vi "Init.vi"(8 "error in (no error)":errorcluster, 9 "ExecCtrlRefs":T1) -> (0 "error out":errorcluster, 3 "UI ExecutionCtrls out":refnum<class "UI ExecutionCtrls.lvclass">)   [LabVIEW 2019, in "UI ExecutionCtrls.lvclass"]
doc: "store control refs for updating the UI\ninit controls"
uses:
  UI ExecutionCtrls.lvclass
  MotionExecutionCtrlRefs.ctl
  UI ExecutionCtrls.lvclass/UI ExecutionCtrls.ctl
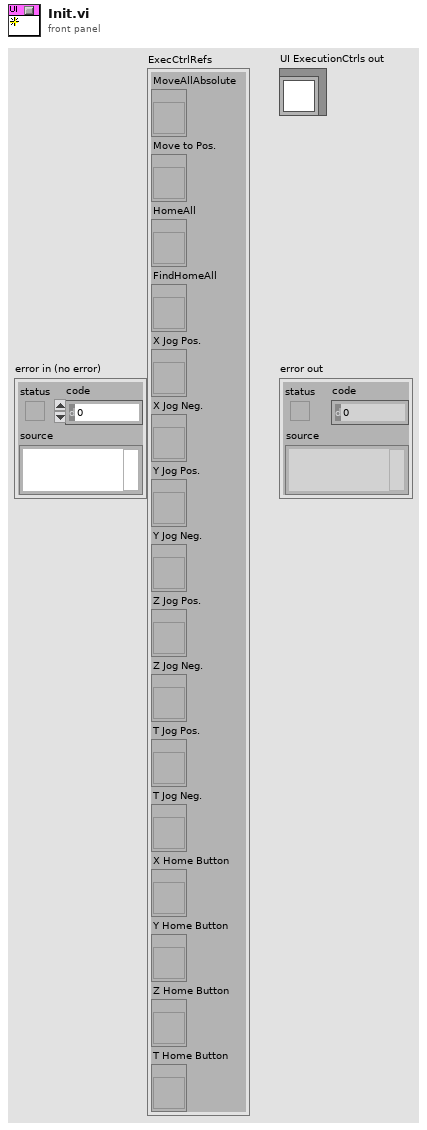
[diagram p1: front panel]
types:
  T1 = typedef "MotionExecutionCtrlRefs.ctl" = cluster{"MoveAllAbsolute":refnum<vi>, "Move to Pos.":refnum<vi>, "HomeAll":refnum<vi>, "FindHomeAll":refnum<vi>, "X Jog Pos.":refnum<vi>, "X Jog Neg.":refnum<vi>, "Y Jog Pos.":refnum<vi>, "Y Jog Neg. ":refnum<vi>, "Z Jog Pos.":refnum<vi>, "Z Jog Neg.":refnum<vi>, "T Jog Pos.":refnum<vi>, "T Jog Neg.":refnum<vi>, "X Home Button":refnum<vi>, "Y Home Button":refnum<vi>, "Z Home Button":refnum<vi>, "T Home Button":refnum<vi>}
  T2 = enum8{"Enabled", "Disabled", "Disabled and Grayed Out"}
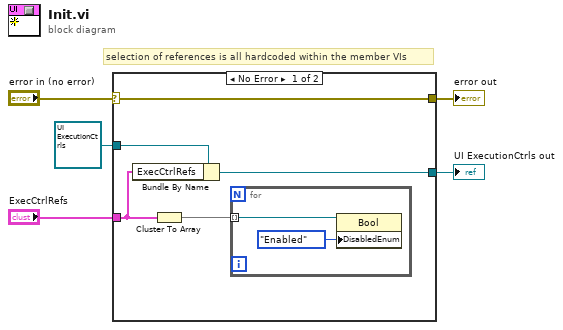
[diagram p0: block diagram]
diagram:
  # "selection of references is all hardcoded within the member VIs"
  n1 = case shown="No Error" "error in (no error)" {
    selector: "error in (no error)" -> [w9 w14]
    tunnel: [w9 w14] -> w4
    tunnel: [w8 w13] -> w2
    tunnel: refnum<class "UI ExecutionCtrls.lvclass"> refnum ("UI ExecutionCtrls in") -> [w10 w13]
    tunnel: "ExecCtrlRefs" -> [w7 _]
    frame No Error {
      n2 = Bundle By Name(cluster=w10, "ExecCtrlRefs"=w7) -> (w8:refnum<class "UI ExecutionCtrls.lvclass">)
      n3 = Cluster To Array(cluster=w7) -> (array=w6:refnum<vi>[])
      n4 = for {
        tunnel: w6 -> [w12] mode=indexing
        n5 = property class="Bool"(reference=w12, "DisabledEnum"=T2."Enabled" ("Disabled")) -> ()  [unwired: 1 in, 2 out]
      }
    }
    frame Error {
    }
  }
  "error out" <- w4
  "UI ExecutionCtrls out" <- w2
